vi "RegisterImagePtr.vi"(8 "error in":errorcluster, 11 "Image Reference In":T1) -> (0 "error out":errorcluster, 2 "ImagePointer":T2 {"ImagePointer" format="%.0x"}, 3 "Image Reference Out":T1)   [LabVIEW 2024, in "OpenLvVision_Image.lvlib" / "DataAccess.lvlib"]
doc: "Provides the image's memory pointer and alignment details."
uses:
  DataAccess.lvlib
  TypeDef/ImagePointer.ctl
  Management/TypeDef/ImageType.ctl
  Management/TypeDef/Image.ctl
  Management/Management.lvlib
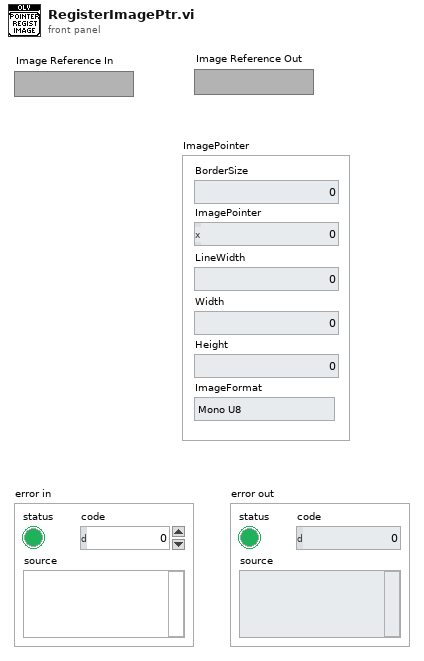
[diagram p1: front panel]
types:
  T1 = typedef "OpenLvVision_Image.lvlib/Management.lvlib/Image.ctl" = refnum<image>
  T2 = typedef "OpenLvVision_Image.lvlib/DataAccess.lvlib/ImagePointer.ctl" = cluster{"BorderSize":i32, "ImagePointer":u64, "LineWidth":i32, "Width":i32, "Height":i32, "ImageFormat":T3}
  T3 = typedef "OpenLvVision_Image.lvlib/Management.lvlib/ImageType.ctl" = enum16{"Mono U8", "Mono U16", "Mono I16", "Mono SGL", "Color U32", "Color U64"}
  T4 = typedef "OpenLvVision_Image.lvlib/DataAccess.lvlib/PixelPointer.ctl" = cluster{"Image Border Size":i32, "Pixel Pointer":u64, "LineWidth":i32, "PixelSize_Bytes":i32, "TransferMaxSize":i32}
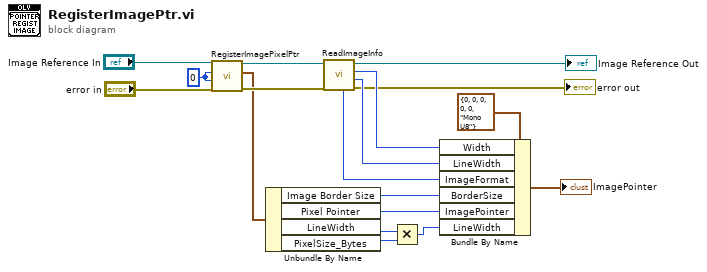
[diagram p0: block diagram]
diagram:
  w18 = 0
  n1 = call "RegisterImagePixelPtr.vi"("error in"="error in", "Y Coordinate"=w18, "X Coordinate"=w18, "Image Reference In"="Image Reference In") -> ("error out"=w17:errorcluster, "PixelPointer"=w11:T4, "Image Reference Out"=w5:T1)  [unwired: 5 in]
  n2 = Unbundle By Name(w11) -> ("Image Border Size"=w10:i32, "Pixel Pointer"=w9:u64, "LineWidth"=w8:i32, "PixelSize_Bytes"=w7:i32)
  n3 = call "ReadImageInfo.vi"("error in"=w17, "Image Reference In"=w5) -> ("error out"=→"error out":errorcluster, "Height"=w13:i32, "Width"=w14:i32, "Image Reference Out"=→"Image Reference Out":T1, "Image Type"=w12:T3)  [unwired: 4 in, 1 out]
  n4 = Multiply(x=w8, y=w7) -> (x*y=w6:i32)
  n5 = Bundle By Name(cluster=T2 {"BorderSize"=0, "ImagePointer"=0, "LineWidth"=0, "Width"=0, "Height"=0, "ImageFormat"=enum."Mono U8"} ("ImagePointer"), "Width"=w14, "LineWidth"=w13, "ImageFormat"=w12, "BorderSize"=w10, "ImagePointer"=w9, "LineWidth"=w6) -> (→"ImagePointer":T2)
